vi "SVFA Power Spectral Density Subset.vi"   [LabVIEW 2017]
doc: "Computes a subset of the power spectral density of <B>scaled signal [EU]</B>. The subset is defined by <B>frequency range</B>. Each block of data corresponds to a single FFT block and has to be passed individually to this VI. Wire data to the <B>scaled signal [EU]</B> input to determine the polymorphic instance to use or manually select the instance."
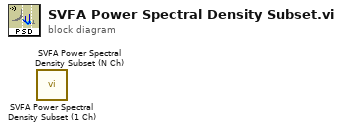
[diagram p0: block diagram]
diagram:
  n1 = call <vilib>:"SVFA Power Spectral Density Subset (1 Ch).vi"() -> ()  [unwired: 14 in, 6 out]
  n2 = call <vilib>:"SVFA Power Spectral Density Subset (N Ch).vi"() -> ()  [unwired: 14 in, 6 out]
